vi "Emit.vi"(8 "error in (no error)":errorcluster, 10 "JSON Token Type":T1, 11 "JSON Lexer in":refnum<class "JSON Lexer.lvclass">) -> (0 "error out":errorcluster, 3 "JSON Lexer out":refnum<class "JSON Lexer.lvclass">)   [LabVIEW 2019, in "JKI JSON Serialization.lvlib" / "JSON Lexer.lvclass"]
doc: "JKI JSON 1.1.10.37\nTomi Maila - JKI\nCopyright (c) 2017, JKI"
uses:
  JSON Lexer.lvclass
  JSON Token Type.ctl
  JSON Lexer.lvclass/JSON Lexer.ctl
  Unicode/UTF-8 String/UTF-8 String.lvclass/UTF-8 String.ctl
  Unicode/UTF-8 String/UTF-8 String.lvclass
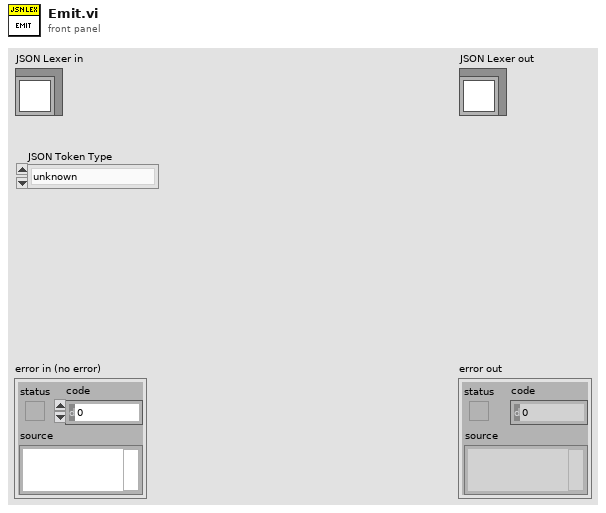
[diagram p1: front panel]
types:
  T1 = typedef "JKI JSON Serialization.lvlib/JSON Lexer.lvclass/JSON Token Type.ctl" = enum32{"unknown", "comma", "end-label", "begin-object", "end-object", "begin-array", "end-array", "quoted-string", "boolean", "exponential-number", "decimal-number", "integer-number", "special-number", "null", "symbol", "whitespace", "EOF"}
  T2 = cluster{"JSON Token Type":T1, "String Subset":string}
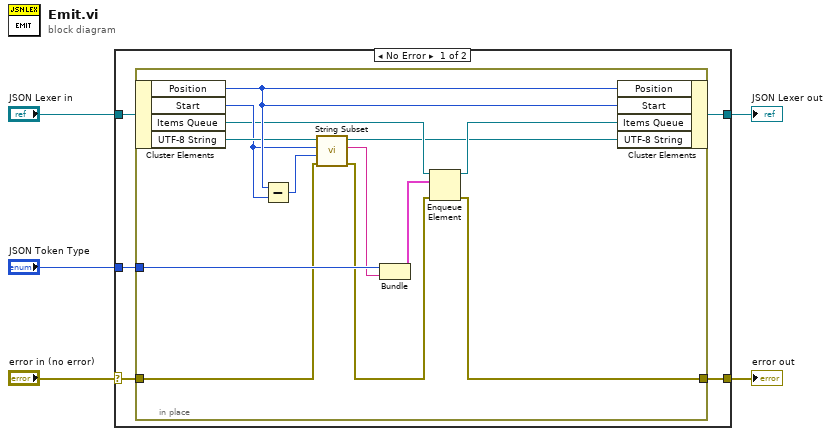
[diagram p0: block diagram]
diagram:
  n1 = case shown="No Error" "error in (no error)" {
    selector: "error in (no error)" -> [w10 w25]
    tunnel: [w9 w25] -> w4
    tunnel: [w7 w24] -> w2
    tunnel: "JSON Lexer in" -> [w6 w24]
    tunnel: "JSON Token Type" -> [w8 _]
    frame No Error {
      n2 = in-place {
        in-place-border: w10 -> [w15]
        in-place-border: [w23] -> w9
        in-place-border: w8 -> [w22]
        n3 = in-place-cluster #1(w6) -> ("Position"=w20:i32, "Start"=w18:i32, "Items Queue"=w13:refnum<queue>, "UTF-8 String"=w19:refnum<class "UTF-8 String.lvclass">)
        n4 = Subtract(x=w20, y=w18) -> (x-y=w17:i32)
        n5 = call "String Subset.vi"("error in (no error)"=w15, "Length in Bytes (0)"=w17, "Byte Offset (0)"=w18, "UTF8 in"=w19) -> ("error out"=w14:errorcluster, "String Subset"=w16:string, "UTF8 out"=w11:refnum<class "UTF-8 String.lvclass">)  [unwired: 5 in]
        n6 = Bundle("JSON Token Type"=w22, "String Subset"=w16) -> (w21:T2)  [unwired: 1 in]
        n7 = Enqueue Element(queue=w13, element=w21, error in (no error)=w14) -> (queue out=w12:refnum<queue>, error out=w23:errorcluster)  [unwired: 1 in, 1 out]
        n8 = in-place-cluster #1("Position"=w20, "Start"=w20, "Items Queue"=w12, "UTF-8 String"=w11) -> (w7:refnum<class "JSON Lexer.lvclass">)
      }
    }
    frame Error {
    }
  }
  "error out" <- w4
  "JSON Lexer out" <- w2
